vi "changeTarget.vi"(8 "error in (no error)":errorcluster, 9 "targetNumber":i16, 10 "interface object in":refnum<k20>, 11 "MotorControllerClass in":refnum<class "MotorControllerClass.lvclass">) -> (0 "error out":errorcluster, 1 "changeTargetRes":u32, 2 "interface object out":refnum<k20>, 3 "MotorControllerClass out":refnum<class "MotorControllerClass.lvclass">)   [LabVIEW 2018, in "MotorControllerClass.lvclass"]
uses:
  BMS/MotorControllerClass.lvclass
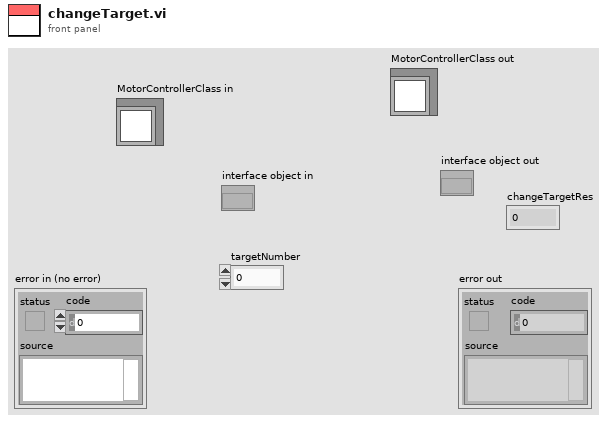
[diagram p1: front panel]
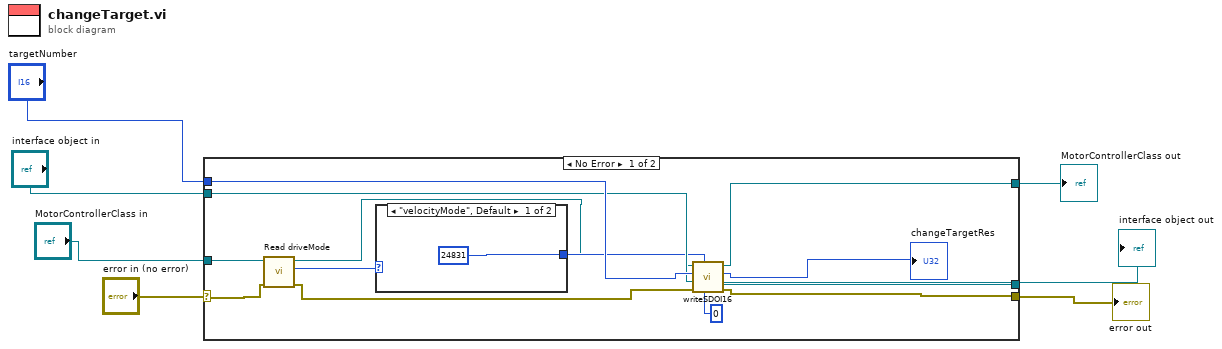
[diagram p0: block diagram]
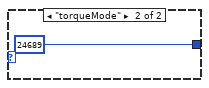
[diagram p2: hidden frame]
diagram:
  n1 = case shown="No Error" "error in (no error)" {
    selector: "error in (no error)" -> [w20 w25]
    tunnel: [w12 w25] -> w6
    tunnel: "targetNumber" -> [w18 _]
    tunnel: "interface object in" -> [w17 w24]
    tunnel: [w10 w24] -> w3
    tunnel: "MotorControllerClass in" -> [w19 w23]
    tunnel: [w9 w23] -> w1
    frame No Error {
      n2 = call-dynamic "Read driveMode.vi"("error in (no error)"=w20, "MotorControllerClass in"=w19) -> ("error out"=w13:errorcluster, "driveMode"=w8:enum16{"velocityMode", "torqueMode", ""}, "MotorControllerClass out"=w14:refnum<class "MotorControllerClass.lvclass">)  [unwired: 7 in]
      n3 = case shown="\"velocityMode\", Default" w8 {
        tunnel: [u16 24831 ("object index") u16 24689 ("object index")] -> w15
        frame "velocityMode", Default {
        }
        frame "torqueMode" {
        }
      }
      n4 = call "writeSDOI16.vi"("object sub-index (0)"=u8 0, "object index"=w15, "error in (no error)"=w13, "interface object in"=w17, "inputNumber"=w18, "MotorControllerClass in"=w14) -> ("error out"=w12:errorcluster, "interface object out"=w10:refnum<k20>, "completion code"=→"changeTargetRes":u32, "MotorControllerClass out"=w9:refnum<class "MotorControllerClass.lvclass">)  [unwired: 2 in]
    }
    frame Error {
    }
  }
  "error out" <- w6
  "interface object out" <- w3
  "MotorControllerClass out" <- w1
